vi "data_packaging_loop.vi"(6 "Message Queues":T1 caption="消息队列", 7 "channel info array":cluster{"Module":string, "Channel":string}[](array[cluster]) caption="通道信息", 8 "error in (no error)":errorcluster caption="错误输入（无错误）", 9 "sampling period (s)":dbl caption="采用周期 (s)", 10 "timestamp":timestamp caption="时间标识", 11 "data queue":refnum<queue> caption="数据队列") -> (0 "error out":errorcluster caption="错误输出")   [LabVIEW 2015]
uses:
  message_queue/all_rt_message_queues.ctl
  message_queue/message_cluster.ctl
  <vilib>/Waveform/WDTOps.llb/WDT Get Final Time Value DBL.vi
  <vilib>/Waveform/WDTOps.llb/WDT Index Channel DBL.vi
  globals/global_all_rt_loop_stop.vi
  message_queue/message_queue.lvlib
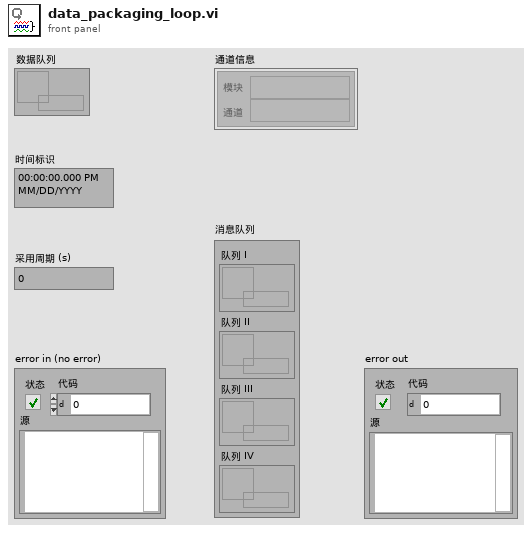
[diagram p1: front panel]
types:
  T1 = typedef "message_queue.lvlib/all_rt_message_queues.ctl" = cluster{"Queue I":refnum<queue>, "Queue II":refnum<queue>, "Queue III":refnum<queue>, "Queue IV":refnum<queue>}
  T2 = enum16{"Initialize", "Acquire Data", "Create Waveform", "Send Waveform"}
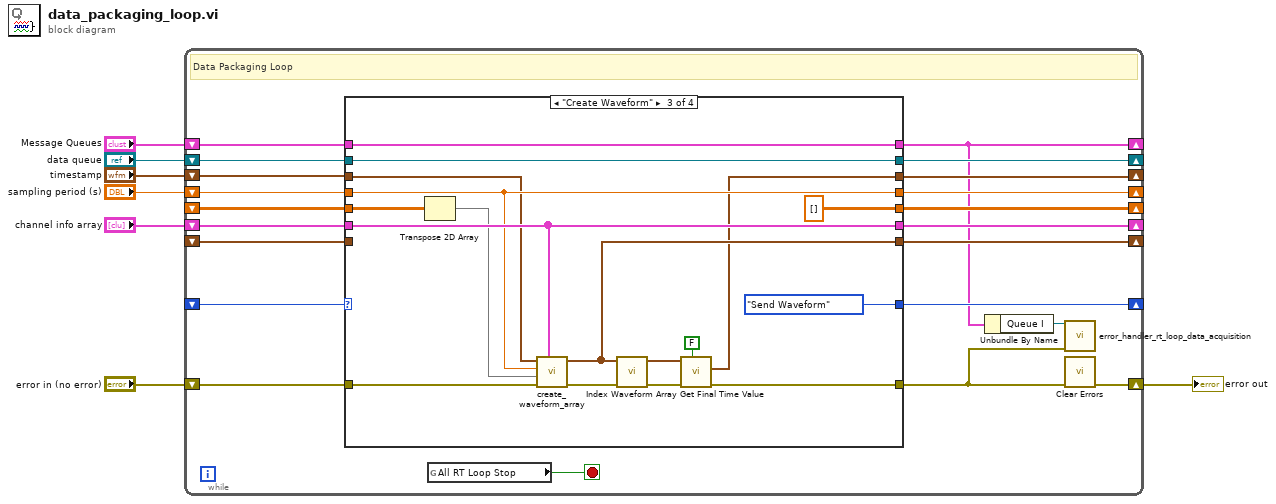
[diagram p0: block diagram]
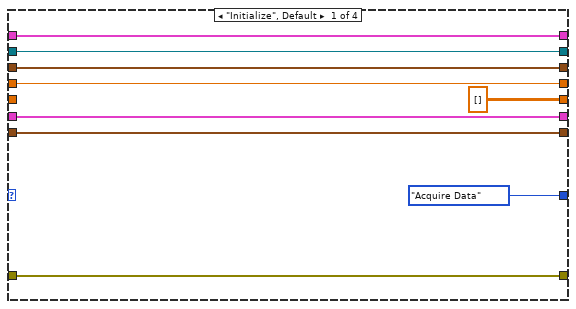
[diagram p2: hidden frame]
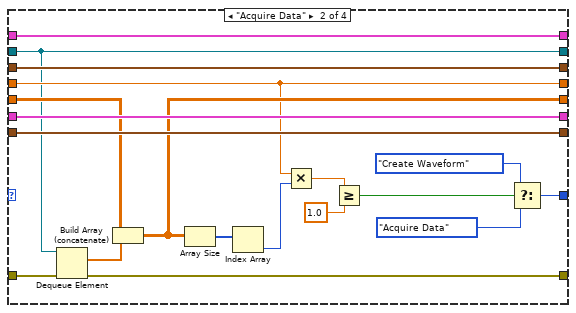
[diagram p3: hidden frame]
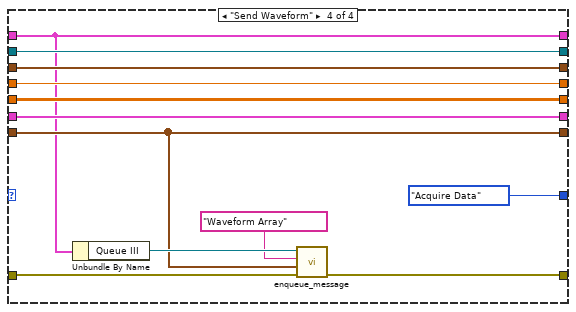
[diagram p4: hidden frame]
diagram:
  n1 = while {
    shift-right: [w28] -> _
    shift-left: "timestamp" -> [w27]
    shift-right: [w21] -> _
    shift-left: _ -> [w22]
    shift-right: [w8] -> _
    shift-left: "Message Queues" -> [w20]
    shift-right: [w19] -> _
    shift-left: _ -> [w18]
    shift-right: [w17] -> w1
    shift-left: "error in (no error)" -> [w25]
    shift-right: [w15] -> _
    shift-left: "data queue" -> [w26]
    shift-right: [w10] -> _
    shift-left: "channel info array" -> [w23]
    shift-right: [w14] -> _
    shift-left: _ -> [w13]
    shift-right: [w9] -> _
    shift-left: "sampling period (s)" -> [w11]
    stop <- w24 stop-if-true
    # "Data Packaging Loop"
    n2 = case shown="\"Create Waveform\"" w22 {
      tunnel: [w32 w53 w57 w79] -> w28
      tunnel: w27 -> [w32 w53 w66 w79]
      tunnel: w23 -> [w33 w52 w69 w80]
      tunnel: w26 -> [w34 w38 w70 w81]
      tunnel: w25 -> [w37 w55 w73 w84]
      tunnel: [w37 w56 w65 w83] -> w16
      tunnel: [T2."Acquire Data" w40 T2."Send Waveform" T2."Acquire Data"] -> w21
      tunnel: w20 -> [w35 w54 w71 w75]
      tunnel: [w35 w54 w71 w75] -> w8
      tunnel: [dbl[][] [] w47 dbl[][] [] w77] -> w19
      tunnel: w18 -> [_ w49 w62 w77]
      tunnel: [w34 w38 w70 w81] -> w15
      tunnel: [w30 w51 w58 w76] -> w14
      tunnel: w13 -> [w30 w51 _ w76]
      tunnel: w11 -> [w31 w45 w67 w78]
      tunnel: [w33 w52 w69 w80] -> w10
      tunnel: [w31 w45 w67 w78] -> w9
      frame "Initialize", Default {
      }
      frame "Acquire Data" {
        n3 = Dequeue Element(queue=w38, error in (no error)=w55) -> (element=w50:dbl[], error out=w56:errorcluster)  [unwired: 1 in, 2 out]
        n4 = Build Array (concatenate)(w49, w50) -> (w47:dbl[][])
        n5 = Array Size(array=w47) -> (size(s)=w48:i32[])
        n6 = Index Array(array=w48) -> (element=w46:i32)  [unwired: 1 in]
        n7 = Multiply(x=w45, y=w46) -> (x*y=w44:dbl)
        n8 = Greater Or Equal?(x=w44, y=1.0) -> (x >= y?=w42:bool)
        n9 = Select(t=T2."Create Waveform", s=w42, f=T2."Acquire Data") -> (s? t:f=w40:T2)
      }
      frame "Create Waveform" {
        n10 = Transpose 2D Array(2D array=w62) -> (transposed array=w68:dbl[][])
        n11 = call "create_waveform_array.vi"("channel info array"=w69, "error in (no error)"=w73, "samples to write"=w68, "sampling period (s)"=w67, "Timestamp"=w66) -> ("error out"=w60:errorcluster, "Waveform Array"=w58:waveform(dbl)[])  [unwired: 5 in]
        n12 = call-poly <vilib>:"Index Waveform Array.vi"("error in (no error)"=w60, "waveform array"=w58) -> ("error out"=w59:errorcluster, "waveform"=w61:waveform(dbl))  [unwired: 8 in]
        n13 = call-poly <vilib>:"Get Final Time Value.vi"("open interval? (T)"=FALSE, "error in (no error)"=w59, "waveform in"=w61) -> ("error out"=w65:errorcluster, "tf"=w57:timestamp)  [unwired: 6 in, 1 out]
      }
      frame "Send Waveform" {
        n14 = Unbundle By Name(w75) -> ("Queue III"=w82:refnum<queue>)
        n15 = call "enqueue_message.vi"("error in (no error)"=w84, "Message Data"=w76, "Message"="Waveform Array", "Message Queue"=w82) -> ("error out"=w83:errorcluster)  [unwired: 6 in, 1 out]
      }
    }
    n16 = global read "global_all_rt_loop_stop.vi" "All RT Loop Stop"() -> (w24:bool)
    n17 = Unbundle By Name(w8) -> ("Queue I"=w12:refnum<queue>)
    n18 = call "error_handler_rt_loop_data_acquisition.vi"("error in (no error)"=w16, "Message Queue"=w12) -> ()  [unwired: 9 in, 1 out]
    n19 = call <vilib>:"Clear Errors.vi"("error in (no error)"=w16) -> ("error out"=w17:errorcluster)  [unwired: 5 in, 1 out]
  }
  "error out" <- w1
